vi "Launch Sensors.vi"(8 "error in (no error)":errorcluster, 11 "DemoMain in":refnum<class "DemoMain.lvclass">) -> (0 "error out":errorcluster, 3 "DemoMain out":refnum<class "DemoMain.lvclass">)   [LabVIEW 2012, in "Win8uiDemo.lvlib" / "DemoMain.lvclass"]
uses:
  DemoMain.lvclass
  Sensor Definition/Sensor.lvclass
  TimerSensor/TimerSensor.lvclass
  TimerSensor/TimerSensorConfig.lvclass
  TimerSensor/TimerView Sensor/Timer Direction.ctl
  <vilib>/ActorFramework/Actor/Actor.lvclass/Actor.ctl
  <vilib>/ActorFramework/Message Enqueuer/Message Enqueuer.lvclass/Message Enqueuer.ctl
  TimerSensor/TimerSensorConfig.lvclass/TimerSensorConfig.ctl
  Sensor Definition/SensorInfo.lvclass
  Sensor Definition/SensorInfo.lvclass/SensorInfo.ctl
  Sensor Definition/Sensor.lvclass/Sensor.ctl
  DemoMain.lvclass/DemoMain.ctl
  TimerSensor/TimerView Sensor/Write Target Time.vi
  TimerSensor/TimerView Sensor/Write Timer Direction.vi
  Sensor Definition/SensorInfo/Write Name.vi
  Sensor Definition/Write Description.vi
  Sensor Definition/SensorInfo/Write Config.vi
  Sensor Definition/Sensor/Write SensorInfo.vi
  Write Sensor Enqueuers.vi
  <vilib>/ActorFramework/Message Enqueuer/Init from Existing Queue.vi
  <vilib>/ActorFramework/Message Enqueuer/Message Enqueuer.lvclass
  <vilib>/ActorFramework/Actor/Actor.lvclass
  TimerSensor/TimerSensor.lvlib
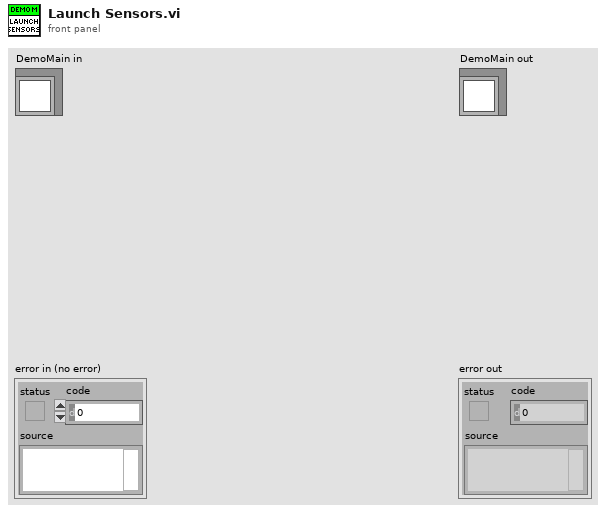
[diagram p1: front panel]
types:
  T1 = typedef "TimerSensor.lvlib/Timer Direction.ctl" = enum16{"Up", "Down"}
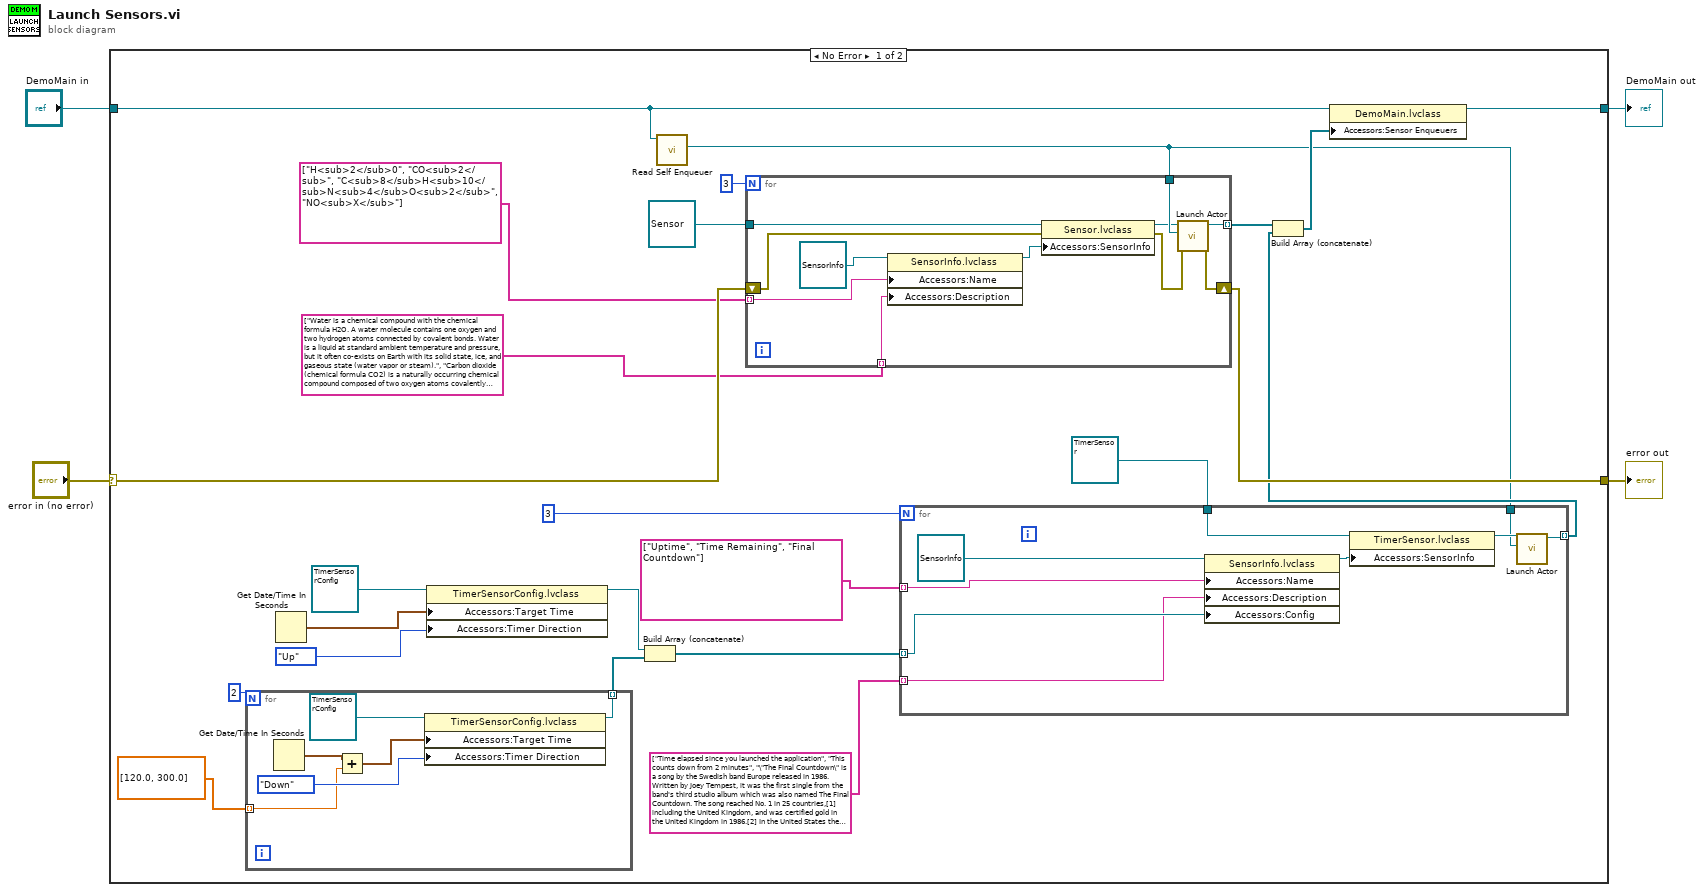
[diagram p0: block diagram]
diagram:
  n1 = case shown="No Error" "error in (no error)" {
    selector: "error in (no error)" -> [w25 w56]
    tunnel: [w24 w56] -> w3
    tunnel: [w28 w55] -> w1
    tunnel: "DemoMain in" -> [w27 w55]
    frame No Error {
      n2 = for {
        N: 2 -> [_]
        tunnel: [w30] -> w11 mode=indexing
        tunnel: dbl[] [120.0, 300.0] -> [w29] mode=indexing
        n3 = Get Date/Time In Seconds() -> (seconds since 1Jan1904=w32:timestamp)
        n4 = Add(x=w32, y=w29) -> (x+y=w31:timestamp)
        n5 = property class="TimerSensorConfig.lvclass"(reference=refnum<class "TimerSensorConfig.lvclass"> refnum ("TimerSensor.lvlib:TimerSensorConfig.lvclass"), "Accessors:Target Time"=w31, "Accessors:Timer Direction"=Timer_Direction."Down" ("Timer Direction")) -> (reference out=w30:refnum<class "TimerSensorConfig.lvclass">)  [unwired: 1 in, 1 out]
      }
      n6 = Get Date/Time In Seconds() -> (seconds since 1Jan1904=w16:timestamp)
      n7 = property class="TimerSensorConfig.lvclass"(reference=refnum<class "TimerSensorConfig.lvclass"> refnum ("TimerSensor.lvlib:TimerSensorConfig.lvclass"), "Accessors:Target Time"=w16, "Accessors:Timer Direction"=Timer_Direction."Up" ("Timer Direction")) -> (reference out=w12:refnum<class "TimerSensorConfig.lvclass">)  [unwired: 1 in, 1 out]
      n8 = Build Array (concatenate)(w12, w11) -> (w10:refnum<class "TimerSensorConfig.lvclass">[])
      n9 = call <vilib>:"Read Self Enqueuer.vi"("Actor"=w27) -> ("Self Enqueuer"=w17:refnum<class "Message Enqueuer.lvclass">)  [unwired: 10 in]
      n10 = for {
        N: 3 -> [_]
        tunnel: refnum<class "Sensor.lvclass"> refnum ("Sensor Definition.lvlib:Sensor.lvclass") -> [w54]
        tunnel: w17 -> [w53]
        tunnel: [w52] -> w23 mode=indexing
        shift-right: [w51] -> w24
        shift-left: w25 -> [w49]
        tunnel: string[] ["H<sub>2</sub>0", "CO<sub>2</sub>", "C<sub>8</sub>H<sub>10</sub>N<sub>4</sub>O<sub>2</sub>", "NO<sub>X</sub>"] -> [w45] mode=indexing
        tunnel: string[] ["Water is a chemical compound with the chemical formula H2O. A water molecule contains one oxygen and two hydrogen atoms connected by covalent bonds. Water is a liquid at standard ambient temperature and pressure, but it often co-exists on Earth with its solid state, ice, and gaseous state (water vapor or steam).", "Carbon dioxide (chemical formula CO2) is a naturally occurring chemical compound composed of two oxygen atoms covalently bonded to a single carbon atom. It is a gas at standard temperature and pressure and exists in Earth's atmosphere in this state, as a trace gas at a concentration of 0.039 per cent by volume.", "Caffeine is a bitter, white crystalline xanthine alkaloid that acts as a stimulant drug. Caffeine is found in varying quantities in the seeds, leaves, and fruit of some plants, where it acts as a natural pesticide that paralyzes and kills certain insects feeding on the plants/", "NOx is a generic term for mono-nitrogen oxides NO and NO2 (nitric oxide and nitrogen dioxide). They are produced from the reaction of nitrogen and oxygen gases in the air during combustion, especially at high temperatures. In areas of high motor vehicle traffic, such as in large cities, the amount of nitrogen oxides emitted into the atmosphere as air pollution can be significant. NOx gases are formed everywhere where there is combustion ? like in an engine."] -> [w44] mode=indexing
        n11 = property class="SensorInfo.lvclass"(reference=refnum<class "SensorInfo.lvclass"> refnum ("Sensor Definition.lvlib:SensorInfo.lvclass"), "Accessors:Name"=w45, "Accessors:Description"=w44) -> (reference out=w46:refnum<class "SensorInfo.lvclass">)  [unwired: 1 in, 1 out]
        n12 = property class="Sensor.lvclass"(reference=w54, error in=w49, "Accessors:SensorInfo"=w46) -> (reference out=w50:refnum<class "Sensor.lvclass">, error out=w48:errorcluster)
        n13 = call <vilib>:"Launch Actor.vi"("error in (no error)"=w48, "Actor-to-Caller Enqueuer"=w53, "Actor"=w50) -> ("error out"=w51:errorcluster, "Caller-To-Actor Enqueuer"=w52:refnum<class "Message Enqueuer.lvclass">)  [unwired: 7 in]
      }
      n14 = for {
        N: 3 -> [_]
        tunnel: refnum<class "TimerSensor.lvclass"> refnum ("TimerSensor.lvlib:TimerSensor.lvclass") -> [w42]
        tunnel: [w39] -> w20 mode=indexing
        tunnel: w17 -> [w38]
        tunnel: w10 -> [w37] mode=indexing
        tunnel: string[] ["Time elapsed since you launched the application", "This counts down from 2 minutes", "\"The Final Countdown\" is a song by the Swedish band Europe released in 1986. Written by Joey Tempest, it was the first single from the band's third studio album which was also named The Final Countdown. The song reached No. 1 in 25 countries,[1] including the United Kingdom, and was certified gold in the United Kingdom in 1986.[2] In the United States the song peaked at No. 8 on the Billboard Hot 100 and 18 on the Billboard Mainstream Rock Tracks chart."] -> [w36] mode=indexing
        tunnel: string[] ["Uptime", "Time Remaining", "Final Countdown"] -> [w35] mode=indexing
        n15 = property class="SensorInfo.lvclass"(reference=refnum<class "SensorInfo.lvclass"> refnum ("Sensor Definition.lvlib:SensorInfo.lvclass"), "Accessors:Name"=w35, "Accessors:Description"=w36, "Accessors:Config"=w37) -> (reference out=w41:refnum<class "SensorInfo.lvclass">)  [unwired: 1 in, 1 out]
        n16 = property class="TimerSensor.lvclass"(reference=w42, "Accessors:SensorInfo"=w41) -> (reference out=w40:refnum<class "TimerSensor.lvclass">)  [unwired: 1 in, 1 out]
        n17 = call <vilib>:"Launch Actor.vi"("Actor-to-Caller Enqueuer"=w38, "Actor"=w40) -> ("Caller-To-Actor Enqueuer"=w39:refnum<class "Message Enqueuer.lvclass">)  [unwired: 8 in, 1 out]
      }
      n18 = Build Array (concatenate)(w23, w20) -> (w18:refnum<class "Message Enqueuer.lvclass">[])
      n19 = property class="DemoMain.lvclass"(reference=w27, "Accessors:Sensor Enqueuers"=w18) -> (reference out=w28:refnum<class "DemoMain.lvclass">)  [unwired: 1 in, 1 out]
    }
    frame Error {
    }
  }
  "error out" <- w3
  "DemoMain out" <- w1
